vi "Helper - BuoyPoints.vi"(7 "Distance":dbl=2.0, 9 "K":dbl, 10 "East":dbl, 11 "North":dbl) -> (0 "NorthOut 2":dbl, 1 "East Out 2":dbl, 2 "NorthOut":dbl, 3 "East Out":dbl)   [LabVIEW 2011]
panel:
  # "2m distance to buoy Default Value\nCan be changed depending on Waypoint precision"
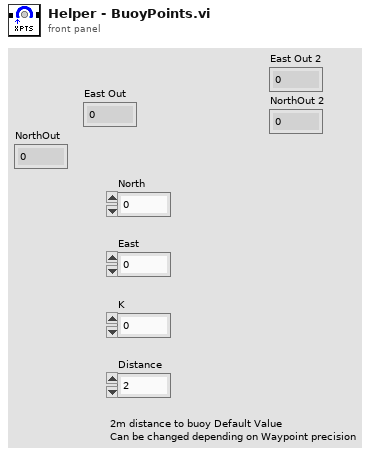
[diagram p1: front panel]
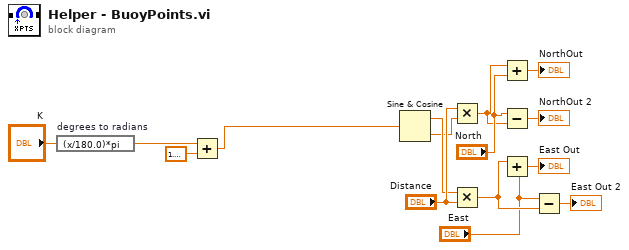
[diagram p0: block diagram]
diagram:
  n1 = expression code="(x/180.0)*pi" "degrees to radians"("K") -> (w14:dbl)
  n2 = Add(x=w14, y=1.5707963267948966) -> (x+y=w5:dbl)
  n3 = Sine & Cosine(0:w5) -> (1:w7:dbl, 2:w6:dbl)
  n4 = Multiply(x="Distance", y=w6) -> (x*y=w1:dbl)
  n5 = Multiply(x=w7, y="Distance") -> (x*y=w4:dbl)
  n6 = Add(x=w1, y="North") -> (x+y=→"NorthOut":dbl)
  n7 = Subtract(x="North", y=w1) -> (x-y=→"NorthOut 2":dbl)
  n8 = Add(x=w4, y="East") -> (x+y=→"East Out":dbl)
  n9 = Subtract(x="East", y=w4) -> (x-y=→"East Out 2":dbl)
